vi "property_write_read_harness.vi"() -> ()   [LabVIEW 2020]
panel:
  out "result":u32
  in  "value":u32
  in  "target":u32
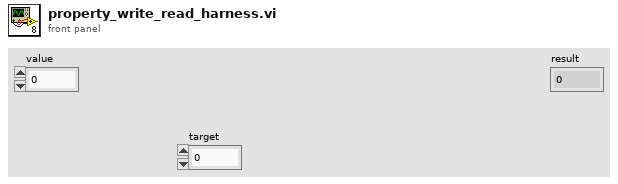
[diagram p1: front panel]
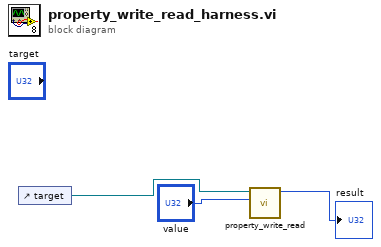
[diagram p0: block diagram]
diagram:
  n1 = control-ref of="target"() -> (w3:refnum<vi>)
  n2 = call "property_write_read.vi"("value"="value", "Digital in"=w3) -> ("result"=→"result":u32)  [unwired: 9 in]
